vi "Set Slot.vi"(8 "error in":errorcluster, 10 "module":refnum<class "Module.lvclass">, 11 "slot ref in":T2 format="%.0x") -> (0 "error out":errorcluster, 3 "slot ref out":T2 format="%.0x")   [LabVIEW 2020, in "Scan Engine Scripting.lvlib"]
doc: "Writes a module configuration for a slot."
uses:
  Scan Engine Scripting.lvlib
  <vilib>/NI VeriStand/Custom Device API/Custom Device Item Ref.ctl
  Modules/Module/Module.lvclass
  Modules.lvlibp/RSI Module/Module Models.ctl
  Modules/NI 9224/NI 9224.lvclass
  Modules.lvlibp/9224/9224.lvclass
  C:/jenkins/workspace/ercat-custom-device_release_20.4/Custom Device Source/Modules.lvlibp/RSI Module/RSI Module.lvclass
  Modules/NI 9228/NI 9228.lvclass
  Modules.lvlibp/9212/9212.lvclass
  Modules/NI 9212/NI 9212.lvclass
  Modules.lvlibp/9213/9213.lvclass
  Modules/NI 9213/NI 9213.lvclass
  Scan Engine Dependencies.llb/Error Strings.vi
  <vilib>/regexp/Match Regular Expression.xnode
  Modules.lvlibp/RSI Module/RSI Module.lvclass
  Custom Device Source/Modules.lvlibp
  Scan Engine Dependencies.llb/Scan Engine Custom Device.lvlib
  Modules/Mode Classes/Mode/Mode.lvclass
  <vilib>/NI VeriStand/Custom Device API/Custom Device API.lvlib
panel:
  in  "module model":T1
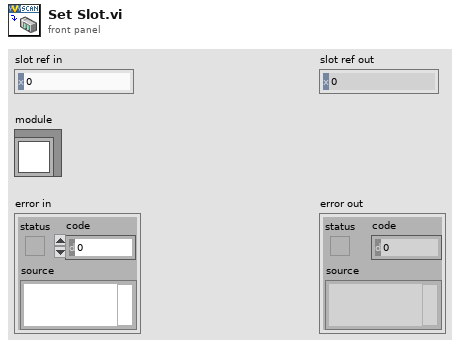
[diagram p1: front panel]
types:
  T1 = typedef "Modules.lvlibp/RSI Module.lvclass/Module Models.ctl" = enum16{"Empty", "NI 9201", "NI 9203", "NI 9205", "NI 9206", "NI 9207", "NI 9208", "NI 9209", "NI 9210", "NI 9211", "NI 9212", "NI 9213", "NI 9214", "NI 9215", "NI 9216", "NI 9217", "NI 9219", "NI 9220", "NI 9221", "NI 9222", "NI 9223", "NI 9224", "NI 9225", "NI 9226", "NI 9227", "NI 9228", "NI 9229", "NI 9233", "NI 9234", "NI 9235", "NI 9236", "NI 9237", "NI 9239", "NI 9242", "NI 9244", "NI 9253", "NI 9263", "NI 9264", "NI 9265", "NI 9266", "NI 9269", "NI 9344", "NI 9350", "NI 9375", "NI 9401", "NI 9402", "NI 9403", "NI 9411", "NI 9421", "NI 9422", "NI 9423", "NI 9425", "NI 9426", "NI 9435", "NI 9436", "NI 9437", "NI 9472", "NI 9474", "NI 9475", "NI 9476", "NI 9477", "NI 9478", "NI 9481", "NI 9482", "NI 9485"}
  T2 = typedef "Custom Device API.lvlib/Custom Device Item Ref.ctl" = u64
  T3 = typedef "Modules.lvlibp/Custom Device API.lvlib/Custom Device Item Ref.ctl" = u64
  T4 = typedef "Modules.lvlibp/RSI Module.lvclass/Slot Settings.ctl" = cluster{"Slot":u32, "EtherCAT?":bool}
  T5 = typedef "Scan Engine Scripting.lvlib/Conversion Time.ctl" = enum16{"High Speed (1k S/s)", "Medium Speed (100 S/s)", "Medium Resolution (50/60Hz Rejection - 12 S/s)", "High Resolution (50/60Hz Rejection - 2 S/s)"}
  T6 = typedef "Scan Engine Scripting.lvlib/Thermocouple Channel.lvclass/Measurement Units.ctl" = enum16{"Raw Volts", "Degrees Kelvin", "Degrees Celsius", "Degrees Fahrenheit", "Degrees Rankine"}
  T7 = typedef "Scan Engine Scripting.lvlib/Thermocouple Channel.lvclass/Thermocouple Type.ctl" = enum16{"J", "K", "T", "E", "R", "S", "N", "B"}
  T8 = typedef "Scan Engine Scripting.lvlib/NI 9212.lvclass/NI 9212 Conversion Time.ctl" = enum16{"High Speed", "Best 60 Hz Rejection", "Best 50 Hz Rejection", "High Resolution"}
  T9 = typedef "Scan Engine Scripting.lvlib/NI 9213.lvclass/NI 9213 Conversion Time.ctl" = enum16{"High Speed", "High Resolution"}
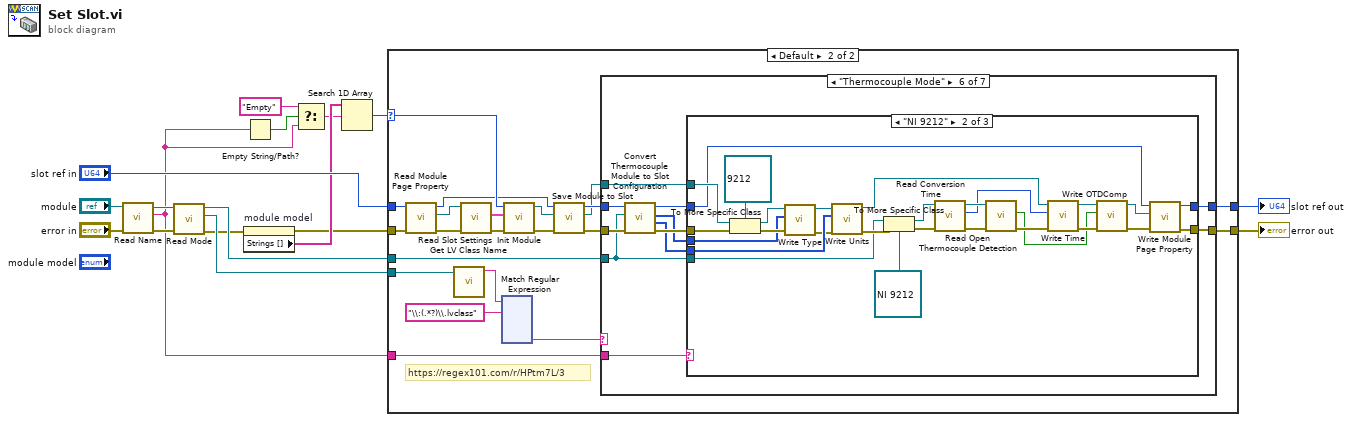
[diagram p0: block diagram]
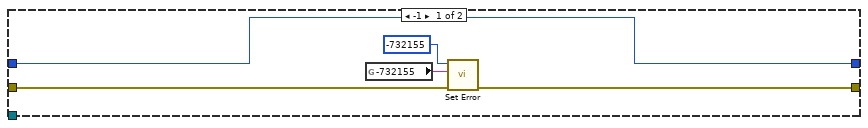
[diagram p2: hidden frame]
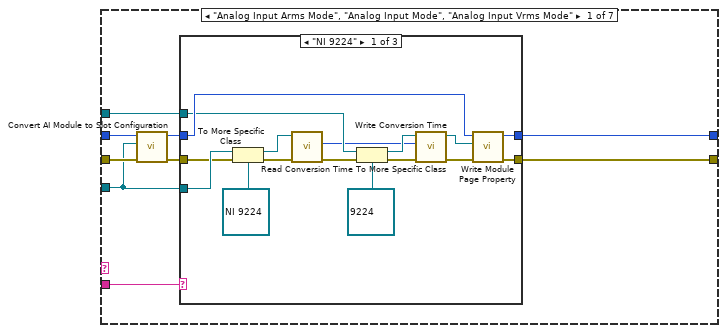
[diagram p3: hidden frame]
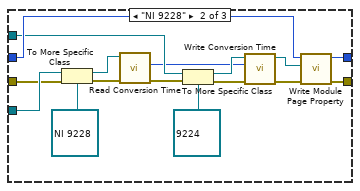
[diagram p4: hidden frame]
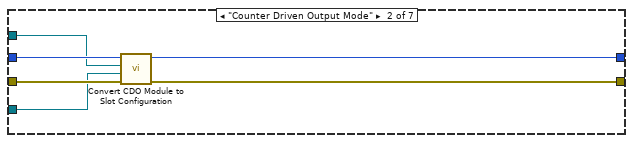
[diagram p6: hidden frame]
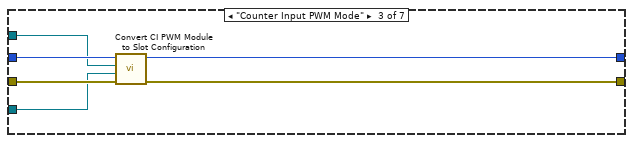
[diagram p7: hidden frame]
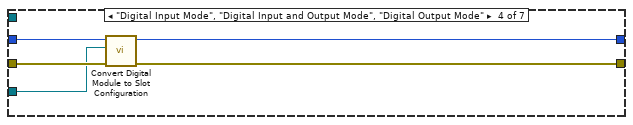
[diagram p8: hidden frame]
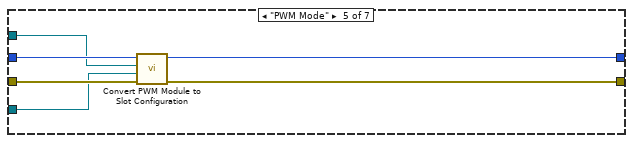
[diagram p9: hidden frame]
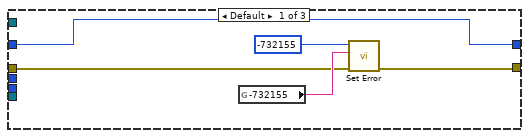
[diagram p10: hidden frame]
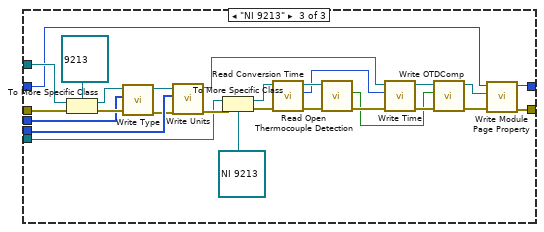
[diagram p11: hidden frame]
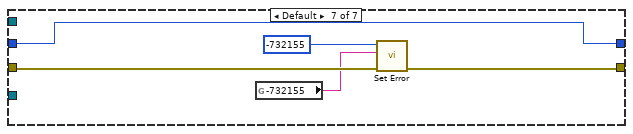
[diagram p12: hidden frame]
diagram:
  n1 = call-dynamic "Read Name.vi"("error in"="error in", "module in"="module") -> ("error out"=w6:errorcluster, "name"=w1:string, "module out"=w5:refnum<class "Module.lvclass">)  [unwired: 7 in]
  n2 = call-dynamic "Read Mode.vi"("error in"=w6, "module in"=w5) -> ("error out"=w2:errorcluster, "mode"=w4:refnum<class "Mode.lvclass">, "module out"=w3:refnum<class "Module.lvclass">)  [unwired: 7 in]
  n3 = property on="module model" class="Enum (strict)"(error in=w2) -> (error out=w12:errorcluster, "Strings []"=w14:string[])  [unwired: 1 in, 1 out]
  n4 = Empty String/Path?(string/path=w1) -> (empty?=w9:bool)
  n5 = Select(t="Empty" ("f"), s=w9, f=w1) -> (s? t:f=w8:string)
  n6 = Search 1D Array(1D array=w14, element=w8) -> (index of element=w13:i32)  [unwired: 1 in]
  n7 = case shown="Default" w13 {
    selector: w13 -> [_ w31]
    tunnel: "slot ref in" -> [w22 w39]
    tunnel: w12 -> [w18 w28]
    tunnel: [w21 w33] -> w16
    tunnel: [w22 w32] -> w15
    tunnel: w4 -> [_ w35]
    tunnel: w3 -> [_ w34]
    tunnel: w1 -> [_ w30]
    frame -1 {
      n8 = global read "Error Strings.vi" "-732155"() -> (w19:string)
      n9 = call "Set Error.vi"("error in (no error)"=w18, "Message"=w19, "Code"=-732155) -> ("error out"=w21:errorcluster)  [unwired: 8 in]
    }
    frame Default {
      # "https://regex101.com/r/HPtm7L/3"
      n10 = call "Read Module Page Property.vi"("error in (no error)"=w28, "Node Ptr In"=w39) -> ("error out"=w43:errorcluster, "RSI Module"=w42:refnum<class "RSI Module.lvclass">, "Node Ptr Out"=w26:T3)  [unwired: 7 in]
      n11 = call <vilib>:"Get LV Class Name.vi"("object"=w35) -> ("class name"=w37:string)  [unwired: 9 in, 1 out]
      n12 = call "Read Slot Settings.vi"("error in (no error)"=w43, "RSI Module in"=w42) -> ("error out"=w41:errorcluster, "Slot Settings"=w40:T4)  [unwired: 7 in, 1 out]
      n13 = xnode "Match Regular Expression"("input string"=w37, "regular expression"="\\:(.*?)\\.lvclass") -> ("submatch 1"=w36:string)  [unwired: 4 in, 5 out]
      n14 = call "Init Module.vi"("error in (no error)"=w41, "Slot Settings"=w40, "Module Model"=w31) -> ("error out"=w29:errorcluster, "RSI Module out"=w24:refnum<class "RSI Module.lvclass">)  [unwired: 7 in]
      n15 = call "Save Module to Slot.vi"("error in"=w29, "RSI module in"=w24, "slot ref in"=w26) -> ("error out"=w27:errorcluster, "RSI module out"=w23:refnum<class "RSI Module.lvclass">, "slot ref out"=w25:T3)  [unwired: 6 in]
      n16 = case shown="\"Thermocouple Mode\"" w36 {
        tunnel: w34 -> [w162 w203 w210 w215 w220 w227 _]
        tunnel: w27 -> [w167 w208 w213 w219 w225 w236 w298]
        tunnel: w23 -> [w161 w204 w209 _ w221 w233 _]
        tunnel: w25 -> [w168 w205 w214 w216 w222 w235 w300]
        tunnel: [w163 w206 w211 w218 w223 w229 w297] -> w33
        tunnel: [w165 w207 w212 w217 w224 w228 w300] -> w32
        tunnel: w30 -> [w160 _ _ _ _ w226 _]
        frame "Analog Input Arms Mode", "Analog Input Mode", "Analog Input Vrms Mode" {
          n17 = call "Convert AI Module to Slot Configuration.vi"("error in"=w167, "module in"=w162, "slot ref in"=w168) -> ("error out"=w164:errorcluster, "slot ref out"=w166:T2)  [unwired: 7 in]
          n18 = case shown="\"NI 9224\"" w160 {
            tunnel: w166 -> [w176 w192 w202]
            tunnel: [w169 w189 w202] -> w165
            tunnel: w164 -> [w183 w199 w201]
            tunnel: [w170 w190 w201] -> w163
            tunnel: w162 -> [w184 w200 _]
            tunnel: w161 -> [w175 w191 _]
            frame "NI 9224" {
              n19 = To More Specific Class(target class=refnum<class "NI 9224.lvclass"> refnum, reference=w184, error in=w183) -> (specific class reference=w174:refnum<class "NI 9224.lvclass">, error out=w173:errorcluster)
              n20 = call-dynamic "Read Conversion Time.vi"("error in"=w173, "NI 9224 in"=w174) -> ("error out"=w172:errorcluster, "conversion time"=w171:T5)  [unwired: 7 in, 1 out]
              n21 = To More Specific Class(target class=refnum<class "9224.lvclass"> refnum ("9224 in"), reference=w175, error in=w172) -> (specific class reference=w181:refnum<class "9224.lvclass">, error out=w180:errorcluster)
              n22 = call-dynamic "Write Conversion Time.vi"("error in"=w180, "Conversion Time"=w171, "9224 in"=w181) -> ("error out"=w179:errorcluster, "9224 out"=w178:refnum<class "9224.lvclass">)  [unwired: 7 in]
              n23 = call "Write Module Page Property.vi"("error in (no error)"=w179, "RSI Module"=w178, "Node Ptr In"=w176) -> ("error out"=w170:errorcluster, "Node Ptr Out"=w169:T3)  [unwired: 6 in, 1 out]
            }
            frame "NI 9228" {
              n24 = To More Specific Class(target class=refnum<class "NI 9228.lvclass"> refnum, reference=w200, error in=w199) -> (specific class reference=w188:refnum<class "NI 9228.lvclass">, error out=w187:errorcluster)
              n25 = call-dynamic "Read Conversion Time.vi"("error in"=w187, "NI 9228 in"=w188) -> ("error out"=w186:errorcluster, "conversion time"=w185:T5)  [unwired: 7 in, 1 out]
              n26 = To More Specific Class(target class=refnum<class "9224.lvclass"> refnum ("9224 in"), reference=w191, error in=w186) -> (specific class reference=w197:refnum<class "9224.lvclass">, error out=w196:errorcluster)
              n27 = call-dynamic "Write Conversion Time.vi"("error in"=w196, "Conversion Time"=w185, "9224 in"=w197) -> ("error out"=w195:errorcluster, "9224 out"=w194:refnum<class "9224.lvclass">)  [unwired: 7 in]
              n28 = call "Write Module Page Property.vi"("error in (no error)"=w195, "RSI Module"=w194, "Node Ptr In"=w192) -> ("error out"=w190:errorcluster, "Node Ptr Out"=w189:T3)  [unwired: 6 in, 1 out]
            }
            frame Default {
            }
          }
        }
        frame "Counter Driven Output Mode" {
          n29 = call "Convert CDO Module to Slot Configuration.vi"("error in"=w208, "module in"=w203, "RSI module in"=w204, "slot ref in"=w205) -> ("error out"=w206:errorcluster, "slot ref out"=w207:T2)  [unwired: 6 in]
        }
        frame "Counter Input PWM Mode" {
          n30 = call "Convert CI PWM Module to Slot Configuration.vi"("error in"=w213, "module"=w210, "RSI module"=w209, "slot ref in"=w214) -> ("error out"=w211:errorcluster, "slot ref out"=w212:T2)  [unwired: 6 in]
        }
        frame "Digital Input Mode", "Digital Input and Output Mode", "Digital Output Mode" {
          n31 = call "Convert Digital Module to Slot Configuration.vi"("error in"=w219, "module"=w215, "slot ref in"=w216) -> ("error out"=w218:errorcluster, "slot ref out"=w217:T2)  [unwired: 7 in]
        }
        frame "PWM Mode" {
          n32 = call "Convert PWM Module to Slot Configuration.vi"("error in"=w225, "module"=w220, "RSI module"=w221, "slot ref in"=w222) -> ("error out"=w223:errorcluster, "slot ref out"=w224:T2)  [unwired: 6 in]
        }
        frame "Thermocouple Mode" {
          n33 = call "Convert Thermocouple Module to Slot Configuration.vi"("error in"=w236, "module"=w227, "slot ref in"=w235) -> ("error out"=w234:errorcluster, "channel measurement units"=w230:T6[], "channel thermocouple types"=w232:T7[], "slot ref out"=w231:T2)  [unwired: 5 in]
          n34 = case shown="\"NI 9212\"" w226 {
            tunnel: w234 -> [w238 w268 w295]
            tunnel: w233 -> [_ w267 w294]
            tunnel: w232 -> [_ w263 w290]
            tunnel: w231 -> [w241 w262 w289]
            tunnel: w230 -> [_ w261 w288]
            tunnel: [w237 w258 w285] -> w229
            tunnel: [w241 w257 w284] -> w228
            tunnel: w227 -> [_ w253 w280]
            frame Default {
              n35 = global read "Error Strings.vi" "-732155"() -> (w239:string)
              n36 = call "Set Error.vi"("error in (no error)"=w238, "Message"=w239, "Code"=-732155) -> ("error out"=w237:errorcluster)  [unwired: 8 in]
            }
            frame "NI 9212" {
              n37 = To More Specific Class(target class=refnum<class "9212.lvclass"> refnum ("9213 in"), reference=w267, error in=w268) -> (specific class reference=w264:refnum<class "9212.lvclass">, error out=w266:errorcluster)
              n38 = call-dynamic "Write Type.vi"("error in (no error)"=w266, "Type"=w263, "9213 in"=w264) -> ("error out"=w260:errorcluster, "9213 out"=w259:refnum<class "9212.lvclass">)  [unwired: 7 in]
              n39 = call-dynamic "Write Units.vi"("error in (no error)"=w260, "Units"=w261, "9213 in"=w259) -> ("error out"=w254:errorcluster, "9213 out"=w256:refnum<class "9212.lvclass">)  [unwired: 7 in]
              n40 = To More Specific Class(target class=refnum<class "NI 9212.lvclass"> refnum ("NI 9212 in"), reference=w253, error in=w254) -> (specific class reference=w251:refnum<class "NI 9212.lvclass">, error out=w252:errorcluster)
              n41 = call-dynamic "Read Conversion Time.vi"("error in"=w252, "NI 9212 in"=w251) -> ("error out"=w249:errorcluster, "conversion time"=w248:T8, "NI 9212 out"=w250:refnum<class "NI 9212.lvclass">)  [unwired: 7 in]
              n42 = call-dynamic "Read Open Thermocouple Detection.vi"("error in"=w249, "NI 9212 in"=w250) -> ("error out"=w247:errorcluster, "open thermocouple detection"=w242:bool)  [unwired: 7 in, 1 out]
              n43 = call-dynamic "Write Time.vi"("error in (no error)"=w247, "Conversion Time"=w248, "9213 in"=w256) -> ("error out"=w246:errorcluster, "9213 out"=w245:refnum<class "9212.lvclass">)  [unwired: 7 in]
              n44 = call-dynamic "Write OTDComp.vi"("error in (no error)"=w246, "OTDComp"=w242, "9212 in"=w245) -> ("error out"=w243:errorcluster, "9212 out"=w244:refnum<class "9212.lvclass">)  [unwired: 7 in]
              n45 = call "Write Module Page Property.vi"("error in (no error)"=w243, "RSI Module"=w244, "Node Ptr In"=w262) -> ("error out"=w258:errorcluster, "Node Ptr Out"=w257:T3)  [unwired: 6 in, 1 out]
            }
            frame "NI 9213" {
              n46 = To More Specific Class(target class=refnum<class "9213.lvclass"> refnum ("9213 in"), reference=w294, error in=w295) -> (specific class reference=w291:refnum<class "9213.lvclass">, error out=w293:errorcluster)
              n47 = call-dynamic "Write Type.vi"("error in (no error)"=w293, "Type"=w290, "9213 in"=w291) -> ("error out"=w287:errorcluster, "9213 out"=w286:refnum<class "9213.lvclass">)  [unwired: 7 in]
              n48 = call-dynamic "Write Units.vi"("error in (no error)"=w287, "Units"=w288, "9213 in"=w286) -> ("error out"=w281:errorcluster, "9213 out"=w283:refnum<class "9213.lvclass">)  [unwired: 7 in]
              n49 = To More Specific Class(target class=refnum<class "NI 9213.lvclass"> refnum ("NI 9212 in"), reference=w280, error in=w281) -> (specific class reference=w278:refnum<class "NI 9213.lvclass">, error out=w279:errorcluster)
              n50 = call-dynamic "Read Conversion Time.vi"("error in"=w279, "NI 9213 in"=w278) -> ("error out"=w276:errorcluster, "conversion time"=w275:T9, "NI 9213 out"=w277:refnum<class "NI 9213.lvclass">)  [unwired: 7 in]
              n51 = call "Read Open Thermocouple Detection.vi"("error in"=w276, "NI 9213 in"=w277) -> ("error out"=w274:errorcluster, "open thermocouple detection"=w269:bool)  [unwired: 7 in, 1 out]
              n52 = call-dynamic "Write Time.vi"("error in (no error)"=w274, "Conversion Time"=w275, "9213 in"=w283) -> ("error out"=w273:errorcluster, "9213 out"=w272:refnum<class "9213.lvclass">)  [unwired: 7 in]
              n53 = call-dynamic "Write OTDComp.vi"("error in (no error)"=w273, "OTDComp"=w269, "9213 in"=w272) -> ("error out"=w270:errorcluster, "9213 out"=w271:refnum<class "9213.lvclass">)  [unwired: 7 in]
              n54 = call "Write Module Page Property.vi"("error in (no error)"=w270, "RSI Module"=w271, "Node Ptr In"=w289) -> ("error out"=w285:errorcluster, "Node Ptr Out"=w284:T3)  [unwired: 6 in, 1 out]
            }
          }
        }
        frame Default {
          n55 = global read "Error Strings.vi" "-732155"() -> (w296:string)
          n56 = call "Set Error.vi"("error in (no error)"=w298, "Message"=w296, "Code"=-732155) -> ("error out"=w297:errorcluster)  [unwired: 8 in]
        }
      }
    }
  }
  "error out" <- w16
  "slot ref out" <- w15
